vi "test Action Update Ramp Rate-errorCase.vi"() -> ()   [LabVIEW 2018, in "Action Update Ramp Rate.lvclass"]
uses:
  Action Update Ramp Rate.lvclass
  Libraries/Thermal Chamber Controller_DQMH/Thermal Chamber Controller_DQMH.lvlib
panel:
  out "TestCase out":refnum<class "Action Update Ramp Rate.lvclass">
  in  "TestCase in":refnum<class "Action Update Ramp Rate.lvclass">
  out "error out":errorcluster
  in  "error in (no error)":errorcluster
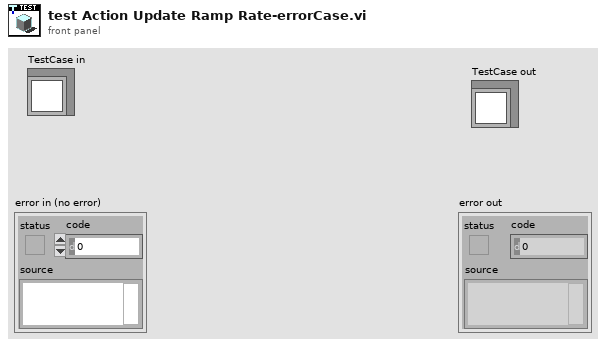
[diagram p1: front panel]
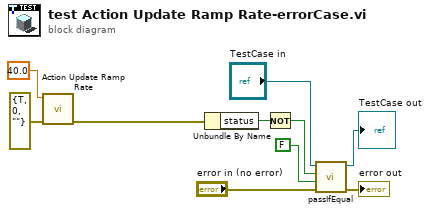
[diagram p0: block diagram]
diagram:
  n1 = call "Action Update Ramp Rate.vi"("error in (no error)"=errorcluster {"status"=TRUE, "code"=0, "source"=""}, "Temperature Ramp Rate"=40.0 ("Temperature Set Point")) -> ("error out"=w6:errorcluster)  [unwired: 9 in]
  n2 = Unbundle By Name(w6) -> ("status"=w7:bool)
  n3 = Not(x=w7) -> (.not. x?=w5:bool)
  n4 = call-dynamic "passIfEqual.vi"("error in (no error)"="error in (no error)", "y"=FALSE, "x"=w5, "TestCase in"="TestCase in") -> ("error out"=→"error out":errorcluster, "TestCase out"=→"TestCase out":refnum<class "Action Update Ramp Rate.lvclass">)  [unwired: 6 in]
